vi "ERIO Globals.vi"() -> ()   [LabVIEW 2017]
doc: "Global variables used in the SteelskyEval RIO demo.\n\nJames Tillett P.E.\nEndeavor Engineering Inc.\nwww.endeavoreng.com"
uses:
  Class EEISysLink/Controls/SL Tag Properties.ctl
  Class EEISysLink/Controls/SL Tag Data Type.ctl
  Class EEISysLink/Controls/SL Tag Interpolation Method.ctl
  Class EEISysLink/Controls/SL Tag Unit of Measure.ctl
  Class EEISysLink/Controls/SL Tag Type.ctl
  Class EEISysLink/EEISysLink.lvclass
panel:
  in  "Enable Tag Property Set":bool
  in  "Tag Properties":T1[](array[typedef])=[{"Class Data Type"=enum."Double", "Name"="ERIO.AlarmThreshold", "Description"="The Amplitude level that will cause an alarm.", "Interpolation Method"=enum."linear", "Unit of Measure"=enum."Volt", "Maximum Interpolation"="10sec", "Role"=enum."Supervisor"}, {"Class Data Type"=enum."Double", "Name"="ERIO.SignalAmplitude", "Description"="Amplitude of the generated signal waveform", "Interpolation Method"=enum."linear", "Unit of Measure"=enum."Volt", "Maximum Interpolation"="10sec", "Role"=enum."Worker"}, {"Class Data Type"=enum."String", "Name"="ERIO.State", "Description"="Current operating stage of conveyor simulation", "Interpolation Method"=enum."linear", "Unit of Measure"=enum."no units", "Maximum Interpolation"="10-sec", "Role"=enum."Worker"}, {"Class Data Type"=enum."Boolean", "Name"="ERIO.EnableSNSAlarm", "Description"="Enable notification message for threshold alarm", "Interpolation Method"=enum."linear", "Unit of Measure"=enum."no units", "Maximum Interpolation"="10sec", "Role"=enum."Supervisor"}, {"Class Data Type"=enum."Boolean", "Name"="ERIO.EnableSNSStageNotifier", "Description"="Enable notification message for stage change", "Interpolation Method"=enum."linear", "Unit of Measure"=enum."no units", "Maximum Interpolation"="10sec", "Role"=enum."Supervisor"}, {"Class Data Type"=enum."Boolean", "Name"="ERIO.EnableSQSNotification", "Description"="Enable notification to SQS queue", "Interpolation Method"=enum."linear", "Unit of Measure"=enum."no units", "Maximum Interpolation"="10sec", "Role"=enum."Supervisor"}, {"Class Data Type"=enum."Boolean", "Name"="ERIO.EnableS3TDMSSignalCapture", "Description"="Enable to send signal capture to S3 file as TDMS", "Interpolation Method"=enum."linear", "Unit of Measure"=enum."no units", "Maximum Interpolation"="10-sec", "Role"=enum."Supervisor"}, {"Class Data Type"=enum."Boolean", "Name"="ERIO.EnableSystemLinkSignalCapture", "Description"="Enable to send signal capture to SystemLink Waveform tag", "Interpolation Method"=enum."linear", "Unit of Measure"=enum."no units", "Maximum Interpolation"="10sec", "Role"=enum."Supervisor"}, {"Class Data Type"=enum."Boolean", "Name"="ERIO.CaptureSignal", "Description"="Request to trigger an amplitude waveform capture or signal", "Interpolation Method"=enum."linear", "Unit of Measure"=enum."no units", "Maximum Interpolation"="10-sec", "Role"=enum."Supervisor"}, {"Class Data Type"=enum."Boolean", "Name"="ERIO.Shutdown", "Description"="Request program shutdown", "Interpolation Method"=enum."linear", "Unit of Measure"=enum."no units", "Maximum Interpolation"="10sec", "Role"=enum."Supervisor"}, {"Class Data Type"=enum."Waveform", "Name"="ERIO.SignalWaveform", "Description"="Contains signal waveform captures", "Interpolation Method"=enum."linear", "Unit of Measure"=enum."Volt", "Maximum Interpolation"="", "Role"=enum."Worker"}, {"Class Data Type"=enum."Boolean", "Name"="ERIO.SignalCaptured", "Description"="Indicate capture signal request has been completed", "Interpolation Method"=enum."linear", "Unit of Measure"=enum."no units", "Maximum Interpolation"="10sec", "Role"=enum."Worker"}, {"Class Data Type"=enum."Double", "Name"="ERIO.StagePercentComplete", "Description"="Percent movement through all 3 stages", "Interpolation Method"=enum."linear", "Unit of Measure"=enum."Percent", "Maximum Interpolation"="10sec", "Role"=enum."Worker"}, {"Class Data Type"=enum."String", "Name"="ERIO.AWSAccessKey", "Description"="Access key for account using the AWS services - Secret key is local to software", "Interpolation Method"=enum."linear", "Unit of Measure"=enum."no units", "Maximum Interpolation"="10sec", "Role"=enum."Supervisor"}, {"Class Data Type"=enum."String", "Name"="ERIO.AWSPhoneNumber", "Description"="Phone number for AWS SNS-SMS interactions", "Interpolation Method"=enum."linear", "Unit of Measure"=enum."no units", "Maximum Interpolation"="10sec", "Role"=enum."Supervisor"}, {"Class Data Type"=enum."Integer", "Name"="ERIO.AWSRegion", "Description"="The AWS datacenter region to use - is enum & strings handled on targets", "Interpolation Method"=enum."linear", "Unit of Measure"=enum."no units", "Maximum Interpolation"="10sec", "Role"=enum."Supervisor"}, {"Class Data Type"=enum."Boolean", "Name"="ERIO.CaptureAvailable", "Description"="Indicate that a new capture has been put in tag", "Interpolation Method"=enum."linear", "Unit of Measure"=enum."no units", "Maximum Interpolation"="10sec", "Role"=enum."Worker"}, {"Class Data Type"=enum."Boolean", "Name"="ERIO.CurrentAlarmState", "Description"="Indicate the current alarm state on target", "Interpolation Method"=enum."linear", "Unit of Measure"=enum."no units", "Maximum Interpolation"="10sec", "Role"=enum."Worker"}, {"Class Data Type"=enum."String", "Name"="ERIO.AWSQueue", "Description"="SQS queue to place notifications", "Interpolation Method"=enum."linear", "Unit of Measure"=enum."Hour", "Maximum Interpolation"="10sec", "Role"=enum."Supervisor"}, {"Class Data Type"=enum."String", "Name"="ERIO.AWSBucket", "Description"="AWS S3 bucket to place TDMS file", "Interpolation Method"=enum."linear", "Unit of Measure"=enum."Hour", "Maximum Interpolation"="10sec", "Role"=enum."Supervisor"}]
  # "Globals used for setup and to reflect SystemLink tag values for development/debug"
  # "TAG VARIABLES SETUP/MANAGEMENT"
  # "Properties used to setup SystemLink tags. \nUsing global with \"set as default\" as a \npersistent tag definition.  Could use a file."
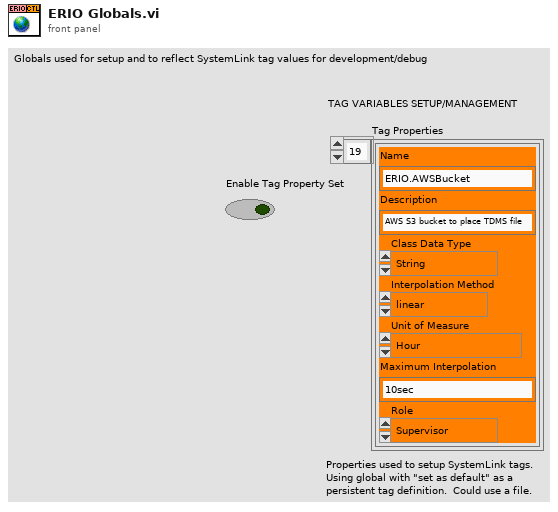
[diagram p1: front panel]
types:
  T1 = typedef "EEISysLink.lvclass/SL Tag Properties.ctl" = cluster{"Class Data Type":T2, "Name":string, "Description":string, "Interpolation Method":T3, "Unit of Measure":T4, "Maximum Interpolation":string, "Role":T5}
  T2 = typedef "EEISysLink.lvclass/SL Tag Data Type.ctl" = enum16{"Double", "Integer", "String", "Boolean", "Waveform"}
  T3 = typedef "EEISysLink.lvclass/SL Tag Interpolation Method.ctl" = enum16{"linear", "pilinear", "step"}
  T4 = typedef "EEISysLink.lvclass/SL Tag Unit of Measure.ctl" = enum16{"no units", "Second", "Hour", "Minute", "Day", "Year", "Month", "Week", "Foot", "Yard", "Meter", "Centimeter", "Inch", "Mile", "Nautical Mile", "Miles per Hour", "Meters per second", "Square meter", "Cubic meter", "Cubic centimeter", "Cubic inch", "Liter", "Gallon", "Gallons dry US", "Gallon UK", "Percent", "Revolutions per minute", "Revolution", "Degree angle", "Astronomical Unit", "Atom", "Atomic mass", "Bar", "Byte", "C (speed of light)", "Curie", "Decibel", "Electron Volt", "Ounce", "Knot", "G", "Grade", "Are", "Hectare", "Faraday", "Franklin", "Gilbert", "Erg", "Lambert", "Maxwell", "Gauss", "Electron mass", "Kilogram force", "Pound force", "Rad", "Centiradian", "Sphere", "Mach", "Fluid Ounces", "Fluid Ounces UK", "Fahrenheit", "Celsius", "Kelvin", "Rankine", "Gram", "Kilogram", "Pound", "Short/US Ton", "Long/UK ton", "Metric ton", "Mole", "Pounds per square inch", "Inches water column", "Torr", "Millitorr", "Millimeter mercury", "Inches mercury", "Bar (2)", "Atmosphere", "Pascal", "Watt", "kiloWatt", "Horsepower", "Kilowatt Hour", "British thermal units", "Millions of BTU", "Ampere", "Candela", "Radian", "Steradian", "Bit", "Hertz", "Newton", "Joule", "Coulomb", "Volt", "Farad", "Ohm", "Siemens", "Weber", "Tesla", "Henry", "Lumen", "Lux", "Becqueral", "Gray", "Sievert", "Katal", "Angstrom", "Light Year", "Parsec", "Point", "Pixel", "Dyne", "Kilogram force (2)", "Pound force (2)", "Rem", "Rutherford", "Roentgen"}
  T5 = typedef "EEISysLink.lvclass/SL Tag Type.ctl" = enum16{"All", "Supervisor", "Worker"}
diagram:
